vi "Mark Initiialized.vi"(8 "error in (no error)":errorcluster, 11 "UniCyRO_Host_Sim in":refnum<class "UniCyRO_Host_Sim.lvclass">) -> (0 "error out":errorcluster, 3 "UniCyRO_Host_Sim out":refnum<class "UniCyRO_Host_Sim.lvclass">)   [LabVIEW 2012, in "UniCyRO.lvlib" / "UniCyRO_Host_Sim.lvclass"]
uses:
  UniCyRO_Host_Sim.lvclass
  UniCyRO_Host_Sim.lvclass/UniCyRO_Host_Sim.ctl
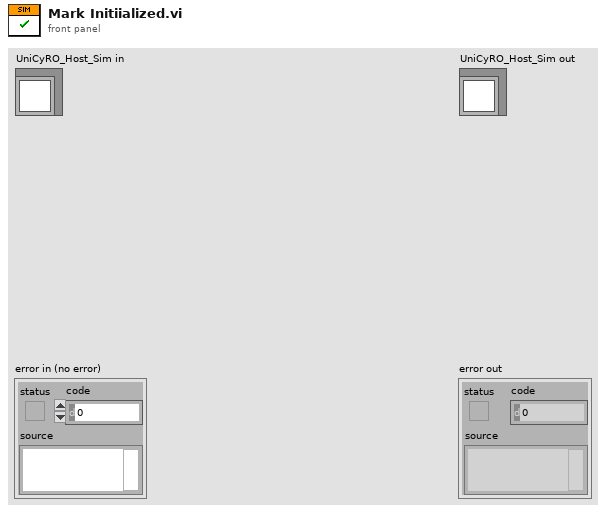
[diagram p1: front panel]
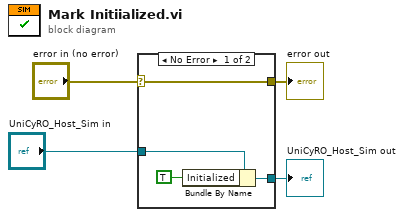
[diagram p0: block diagram]
diagram:
  n1 = case shown="No Error" "error in (no error)" {
    selector: "error in (no error)" -> [w8 w10]
    tunnel: [w8 w10] -> w3
    tunnel: [w5 w9] -> w1
    tunnel: "UniCyRO_Host_Sim in" -> [w6 w9]
    frame No Error {
      n2 = Bundle By Name(cluster=w6, "Initialized"=TRUE) -> (w5:refnum<class "UniCyRO_Host_Sim.lvclass">)
    }
    frame Error {
    }
  }
  "error out" <- w3
  "UniCyRO_Host_Sim out" <- w1
